vi "RSZVB Set Limit Line TTL Out Pass 1(2).vi"(7 "TTL Output (F: Off)":bool, 8 "error in (no error)":errorcluster {"code" format="%.0x"}, 9 "Output No (1)":i32=1, 10 "Channel (Trace) (1)":i32=1, 11 "VISA session":refnum<visa-resource-name>) -> (0 "error out":errorcluster {"code" format="%.0x"}, 3 "dup VISA session":refnum<visa-resource-name>)   [LabVIEW 2011]
doc: "This VI switches the TTL pass/fail signals on or off. The signals are applied to the USER CONTROL connector as long as the active trace <Ch/Tr> is within limits. \n\nRemote-control command(s):\nCALCulate<Ch/Tr>:LIMit:TTLout<Output_no>[:STATe] <Boolean>"
panel:
  # "On\nOff"
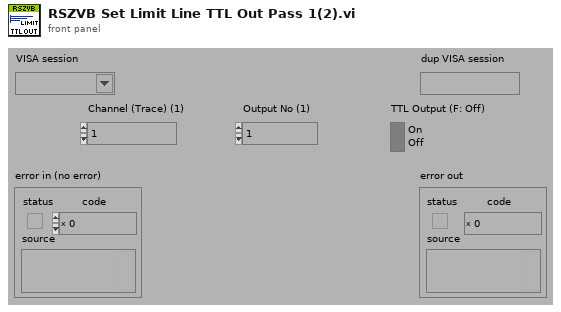
[diagram p1: front panel]
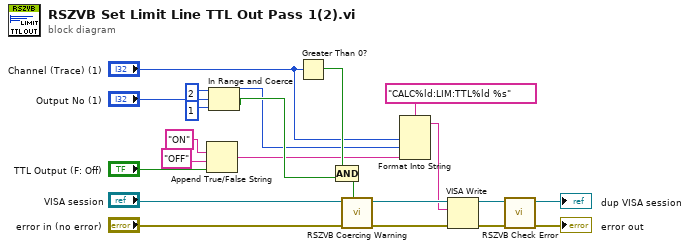
[diagram p0: block diagram]
diagram:
  n1 = Append True/False String(1:"TTL Output (F: Off)", 2:"OFF", 3:"ON") -> (0:w8:string)  [unwired: 1 in]
  n2 = In Range and Coerce(upper limit=2, x="Output No (1)", lower limit=1) -> (coerced(x)=w9:i32, In Range?=w10:bool)
  n3 = Greater Than 0?(x="Channel (Trace) (1)") -> (x > 0?=w15:bool)
  n4 = Compound Arithmetic op=AND(w15, w10) -> (w17:bool)
  n5 = call "RSZVB Coercing Warning.vi"("In Range?"=w17, "error in (no error)"="error in (no error)", "VISA session"="VISA session") -> ("error out"=w20:errorcluster, "dup VISA session"=w21:refnum<visa-resource-name>)  [unwired: 7 in]
  n6 = Format Into String(format string="CALC%ld:LIM:TTL%ld %s", "Channel (Trace) (1)", w9, w8) -> (resulting string=w16:string)  [unwired: 2 in, 1 out]
  n7 = VISA Write(VISA resource name=w21, write buffer=w16, error in (no error)=w20) -> (VISA resource name out=w18:refnum<visa-resource-name>, error out=w19:errorcluster)  [unwired: 1 out]
  n8 = call "RSZVB Check Error.vi"("error in (no error)"=w19, "VISA session"=w18) -> ("error out"=→"error out":errorcluster, "dup VISA session"=→"dup VISA session":refnum<visa-resource-name>)  [unwired: 8 in]
